vi "NumericArrayToString.vi"(11 "Array In":dbl[][](array[numeric])) -> (3 "String Out":string)   [LabVIEW 2017]
doc: "SciScan 1.2 160622"
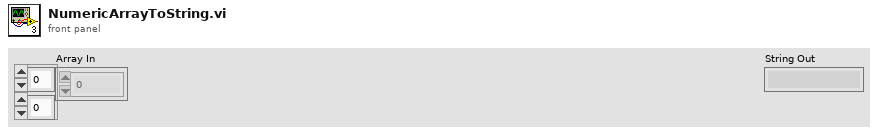
[diagram p1: front panel]
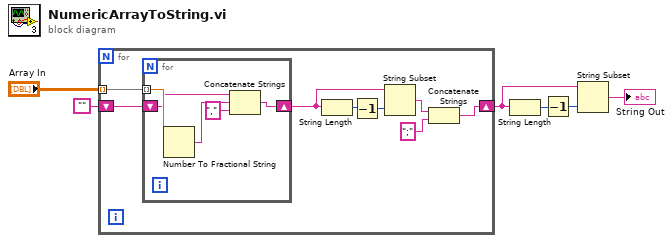
[diagram p0: block diagram]
diagram:
  n1 = for {
    tunnel: "Array In" -> [w14] mode=indexing
    shift-right: [w11] -> w2
    shift-left: "" -> [w13]
    n2 = for {
      tunnel: w14 -> [w19] mode=indexing
      shift-right: [w16] -> w10
      shift-left: w13 -> [w15]
      n3 = Number To Fractional String(number=w19) -> (F-format string=w18:string)  [unwired: 3 in]
      n4 = Concatenate Strings(w15, w18, "," ("string")) -> (w16:string)
    }
    n5 = String Length(string=w10) -> (length=w9:i32)
    n6 = Decrement(x=w9) -> (x-1=w8:i32)
    n7 = String Subset(string=w10, length (rest)=w8) -> (substring=w7:string)  [unwired: 1 in]
    n8 = Concatenate Strings(w7, ";" ("string")) -> (w11:string)
  }
  n9 = String Length(string=w2) -> (length=w3:i32)
  n10 = Decrement(x=w3) -> (x-1=w4:i32)
  n11 = String Subset(string=w2, length (rest)=w4) -> (substring=→"String Out":string)  [unwired: 1 in]
